vi "playing with digital WF create.vi"() -> ()   [LabVIEW 2013]
uses:
  <vilib>/Waveform/DWDTOps.llb/DWDT Boolean Array to Digital.vi
panel:
  out "Digital Waveform Graph":digitalwaveform(graph)
  out "digital waveform":digitalwaveform(waveform)={"t0"=timestamp(0 s since 1904-01-01), "dt"=0.0, "Y"={"transitions"=[], "data"=[]}, "error"={"status"=FALSE, "code"=37421928, "source"=""}}
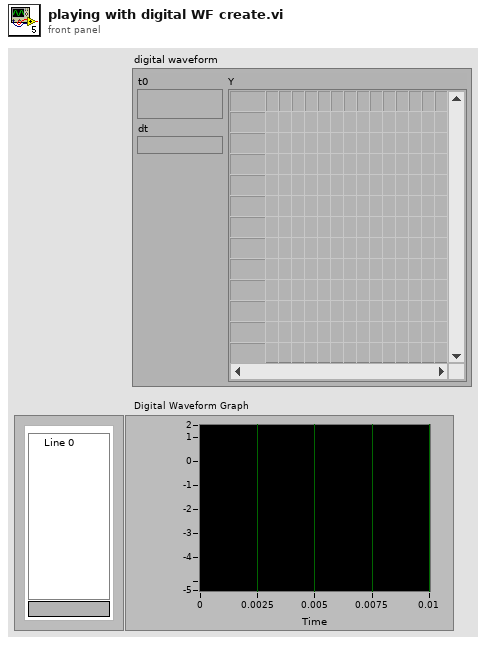
[diagram p1: front panel]
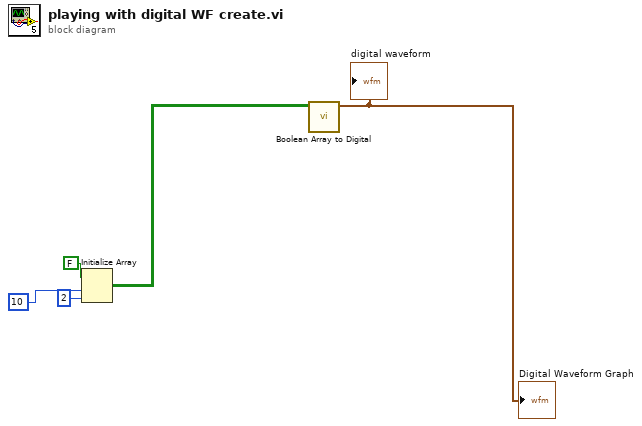
[diagram p0: block diagram]
diagram:
  n1 = Initialize Array(FALSE, 10 ("dimension size"), 2 ("dimension size")) -> (w1:bool[][])
  n2 = call-poly <vilib>:"Boolean Array to Digital.vi"("boolean array"=w1) -> ("digital waveform"=→"digital waveform" →"Digital Waveform Graph":digitalwaveform)  [unwired: 9 in, 1 out]
